vi "Simple Square Root Scaling.vi"(1 "Turret":dbl) -> (0 "Scaled Value":dbl)   [LabVIEW 2019]
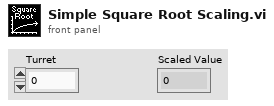
[diagram p1: front panel]
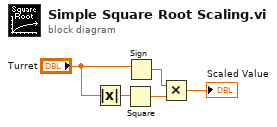
[diagram p0: block diagram]
diagram:
  n1 = Absolute Value(x="Turret") -> (abs(x)=w4:dbl)
  n2 = Square(x=w4) -> (x^2=w3:dbl)
  n3 = Sign(1:"Turret") -> (0:w5:dbl)
  n4 = Multiply(x=w5, y=w3) -> (x*y=→"Scaled Value":dbl)
